vi "FP behavior P-Wall.vi"(1 "Behavior\nVelocity":dbl=20.0, 2 "Activate?":bool=TRUE, 3 "IR Sensors":T1(array[cluster])) -> (0 "P-Wall Array":dbl[](array[numeric]))   [LabVIEW 2014]
doc: "This vi creates a array based upon the value of the PBow IR sensor reading."
uses:
  <vilib>/addons/control/pid/pid.llb/PID (DBL).vi
  <vilib>/addons/control/pid/NI_PID_pid.lvlib
panel:
  out "HPort Setpoint":dbl=40.0 format="%#_13g"
  out "Half-Port\nSensor":string
  out "Port Setpoint":dbl=40.0 format="%#_13g"
  out "steer":dbl format="%.2f"
  out "Port Side Sensor":string
  out "Waveform Graph":cluster{dbl, dbl, dbl[]}(graph)
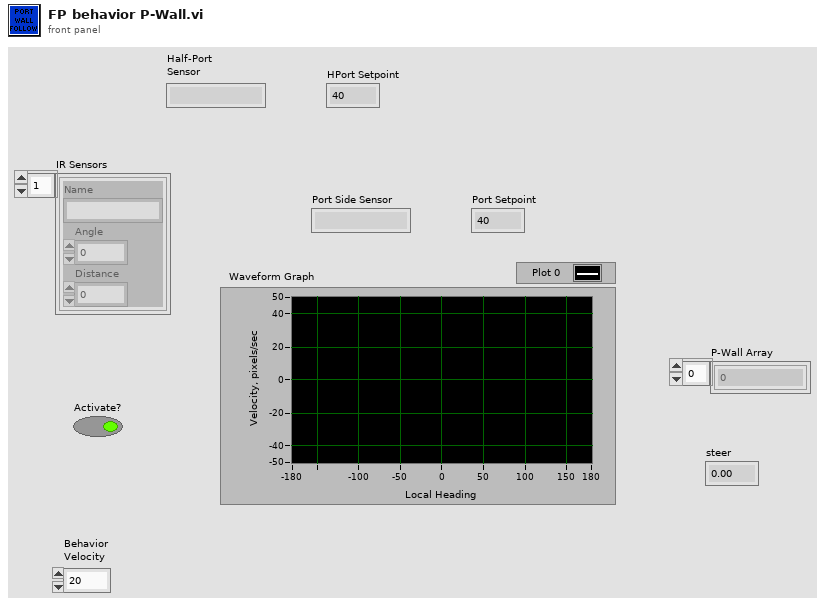
[diagram p1: front panel]
types:
  T1 = cluster{"Name":string, "Angle":dbl, "Distance":dbl}[]
  T2 = cluster{"proportional gain (Kc)":dbl, "integral time (Ti, min)":dbl, "derivative time (Td, min)":dbl}
  T3 = cluster{"Name":string, "Angle":dbl, "Distance":dbl}
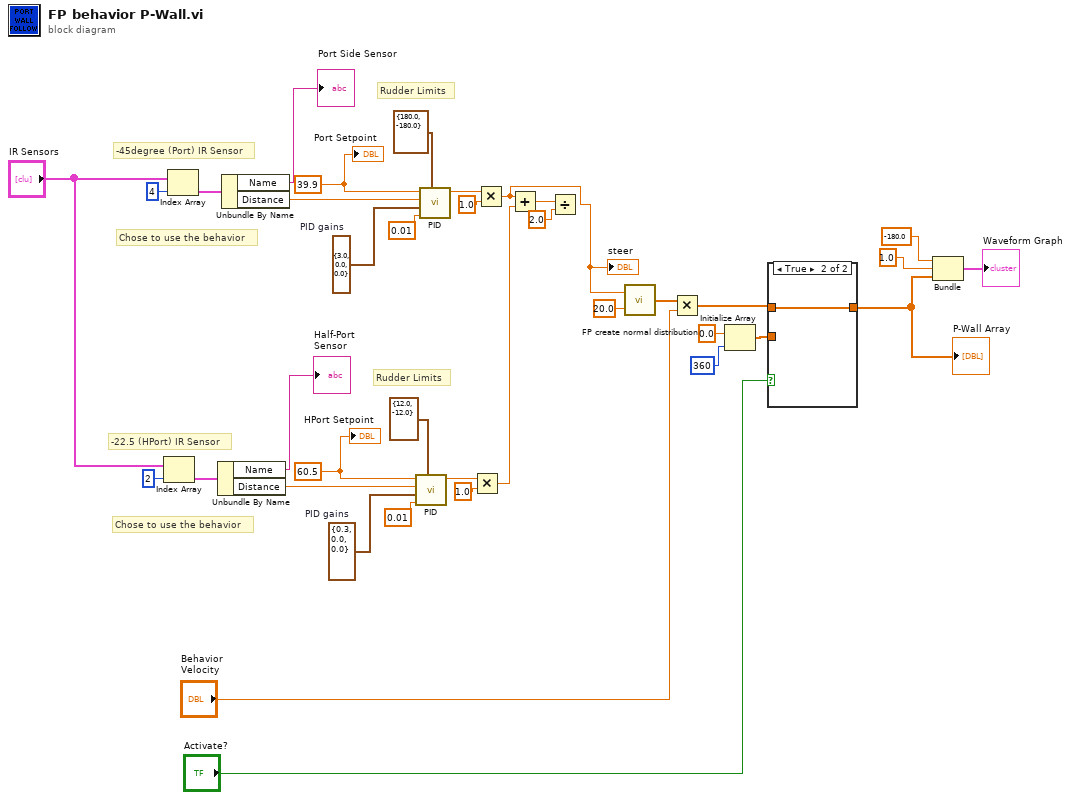
[diagram p0: block diagram]
diagram:
  w2 = 60.5 ("Port Setpoint")
  w3 = 39.9 ("Port Setpoint")
  w9 = T2 {"proportional gain (Kc)"=0.3, "integral time (Ti, min)"=0.0, "derivative time (Td, min)"=0.0}  # PID gains
  w22 = T2 {"proportional gain (Kc)"=3.0, "integral time (Ti, min)"=0.0, "derivative time (Td, min)"=0.0}  # PID gains
  # "-22.5 (HPort) IR Sensor"
  # "-45degree (Port) IR Sensor"
  # "Rudder Limits"
  # "Chose to use the behavior"
  # "Rudder Limits"
  # "Chose to use the behavior"
  n1 = Index Array(array="IR Sensors", index=2) -> (element=w15:T3)
  n2 = Index Array(array="IR Sensors", index=4) -> (element=w28:T3)
  n3 = Unbundle By Name(w15) -> ("Name"=→"Half-Port\nSensor":string, "Distance"=w8:dbl)
  n4 = Unbundle By Name(w28) -> ("Name"=→"Port Side Sensor":string, "Distance"=w21:dbl)
  n5 = call-poly <vilib>:"PID.vi"("output range"=cluster{"output high":dbl, "output low":dbl} {"output high"=12.0, "output low"=-12.0}, "dt (s)"=0.01, "PID gains"=w9, "process variable"=w8, "setpoint"=w2) -> ("output"=w12:dbl)  [unwired: 5 in, 1 out]
  n6 = call-poly <vilib>:"PID.vi"("output range"=cluster{"output high":dbl, "output low":dbl} {"output high"=180.0, "output low"=-180.0}, "dt (s)"=0.01, "PID gains"=w22, "process variable"=w21, "setpoint"=w3) -> ("output"=w25:dbl)  [unwired: 5 in, 1 out]
  n7 = Multiply(x=w12, y=1.0) -> (x*y=w6:dbl)
  n8 = Multiply(x=w25, y=1.0) -> (x*y=w1:dbl)
  "steer" <- w1
  n9 = Add(x=w1, y=w6) -> (x+y=w4:dbl)
  n10 = Divide(x=w4, y=2.0) -> ()  [unwired: 1 out]
  n11 = call "FP create normal distribution.vi"("std (Normal)"=20.0, "mean"=w1) -> ("ACT array"=w20:dbl[])
  n12 = Multiply(x=w20, y="Behavior\nVelocity") -> (x*y=w19:dbl[])
  n13 = Initialize Array(0.0 ("element"), 360 ("dimension size")) -> (w31:dbl[])
  n14 = case shown="True" "Activate?" {
    tunnel: w31 -> [w38 _]
    tunnel: w19 -> [_ w39]
    tunnel: [w38 w39] -> w30
    frame False {
    }
    frame True {
    }
  }
  "P-Wall Array" <- w30
  n15 = Bundle(-180.0, 1.0, w30) -> (→"Waveform Graph":cluster{dbl, dbl, dbl[]})  [unwired: 1 in]
  "Port Setpoint" <- w3
  "HPort Setpoint" <- w2
